vi "Actor Template-Core_Initialize.vi"(0 "Initialization Sequence":string, 5 "FTW Actor Instance Configuration":string, 11 "error in (no error)":errorcluster) -> (4 "Actor Template-Core out":refnum<class "Actor Template-Core.lvclass">, 6 "Incoming Requests":refnum<event-registration>, 8 "Local Messages":refnum<event-registration>, 10 "Refresh Period":dbl, 15 "error out":errorcluster)   [LabVIEW 2013, in "Actor Template-Core.lvclass"]
uses:
  Actor Template-Core.lvclass
  source/actor/Message/Request/FTW-Message-IncomingRequest.lvclass
  source/actor/Message/Base/FTW-Message.lvclass
  Actor Template-Core.lvclass/Actor Template-Core.ctl
  source/JSON/FTW-JSON-Core-LibraryError.vi
  source/Error/FTW-ERR-NoErrorConstant.vi
  source/JSON/FTW-JSON-Core-LibraryFilepath.vi
  source/Reflection/FTW-Reflection-Type.vi
  source/Error/FTW-ERR-ThrowError.vi
  source/Error/FTW-ERR-ThrowGenericError.vi
  source/JSON/FTW-JSON-Core-GetFlattenedValue.vi
  source/CodeGen/JSON Deserialize/FTW-JSON-Deserialize.xnode
  source/JSON/FTW-JSON-Native-GetFlattenedValue.vi
  source/JSON/FTW-JSON-Validate.vi
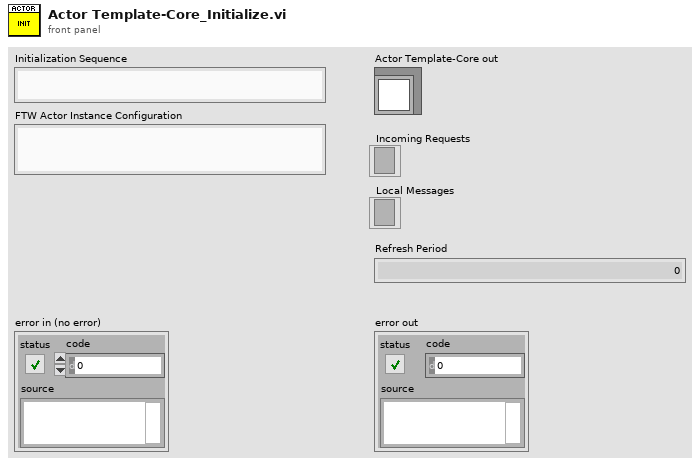
[diagram p1: front panel]
types:
  T1 = cluster{"My Data":bool, "Publisher URI":string, "Subscriber URIs":string, "Refresh Period":dbl}
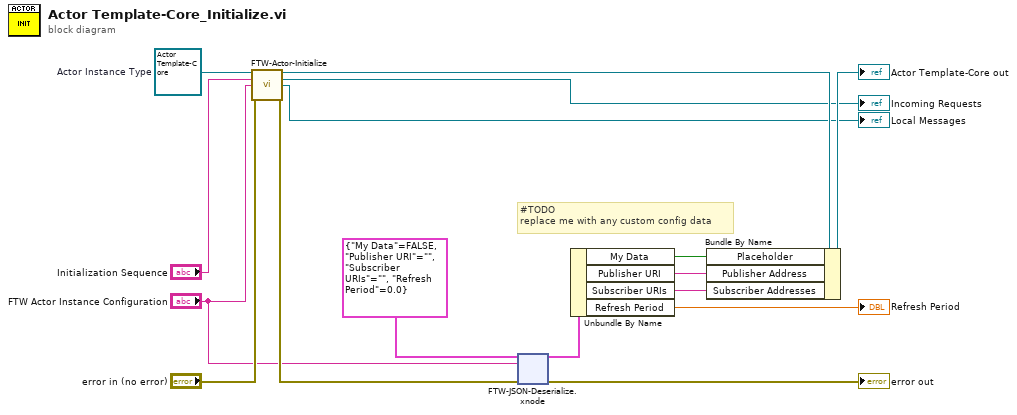
[diagram p0: block diagram]
diagram:
  w16 = refnum<class "Actor Template-Core.lvclass"> refnum  # Actor Instance Type
  # "#TODO\nreplace me with any custom config data"
  n1 = call-dynamic "FTW-Actor-Initialize.vi"("FTW Actor Instance Type"=w16, "Initialization Job Sequence"="Initialization Sequence", "Actor Instance Configuration"="FTW Actor Instance Configuration", "error in"="error in (no error)") -> ("FTW Actor Instance"=w10:refnum<class "Actor Template-Core.lvclass">, "Incoming Requests"=→"Incoming Requests":refnum<event-registration>, "Local Messages"=→"Local Messages":refnum<event-registration>, "error out"=w8:errorcluster)  [unwired: 8 in]
  n2 = xnode "FTW-JSON-Deserialize.xnode"("Type and Defaults"=T1 {"My Data"=FALSE, "Publisher URI"="", "Subscriber URIs"="", "Refresh Period"=0.0}, "JSON String"="FTW Actor Instance Configuration", "error in"=w8) -> ("Values"=w12:T1, "error out"=→"error out":errorcluster)
  n3 = Unbundle By Name(w12) -> ("My Data"=w11:bool, "Publisher URI"=w3:string, "Subscriber URIs"=w2:string, "Refresh Period"=→"Refresh Period":dbl)
  n4 = Bundle By Name(cluster=w10, "Placeholder"=w11, "Publisher Address"=w3, "Subscriber Addresses"=w2) -> (→"Actor Template-Core out":refnum<class "Actor Template-Core.lvclass">)
